vi "Set Sender.vi"(10 "Sender":refnum<class "Sender.lvclass">, 11 "No Op Msg in":refnum<class "No Op Msg.lvclass">) -> (3 "No Op Msg out":refnum<class "No Op Msg.lvclass">)   [LabVIEW 2020, in "jettl.lvlib" / "No Op Msg.lvlib" / "No Op Msg.lvclass"]
uses:
  No Op Msg.lvclass
  Sender/Sender/Sender.lvclass
  No Op Msg.lvclass/No Op Msg.ctl
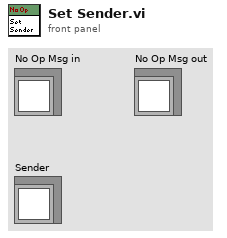
[diagram p1: front panel]
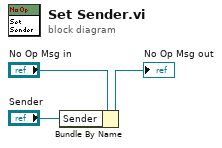
[diagram p0: block diagram]
diagram:
  n1 = Bundle By Name(cluster="No Op Msg in", "Sender"="Sender") -> (→"No Op Msg out":refnum<class "No Op Msg.lvclass">)
